vi "Scripted VI Path.vi"(7 "Terminal Descriptor":T1) -> (2 "Invalid?":bool, 3 "appended path":path)   [LabVIEW 2020, in "Parallel Diagram Block.xnode"]
uses:
  Parallel Diagram Block.xnode
  Parallel Block/Terminal Descriptor.ctl
  Parallel Block/Direction.ctl
  Parallel Block/Value Type.ctl
  Parallel Block/Terminal Type.ctl
  Parallel Block/Parallel Block.lvlib
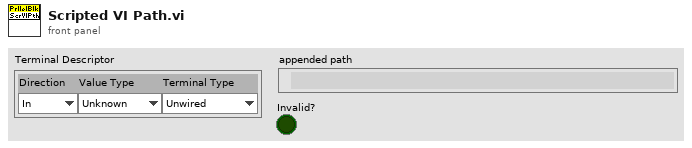
[diagram p1: front panel]
types:
  T1 = typedef "Parallel Block.lvlib/Terminal Descriptor.ctl" = cluster{"Direction":T2, "Value Type":T3, "Terminal Type":T4}
  T2 = typedef "Parallel Block.lvlib/Direction.ctl" = enum16{"In", "Out"}
  T3 = typedef "Parallel Block.lvlib/Value Type.ctl" = enum16{"Unknown", "Bool", "U8", "U16", "U32", "U64", "I8", "I16", "I32", "I64", "SGL", "DBL", "CSG", "CDB", "CDBWfm", "String", "DBLWfm"}
  T4 = typedef "Parallel Block.lvlib/Terminal Type.ctl" = enum16{"Unwired", "Connection", "Value", "Control Ref"}
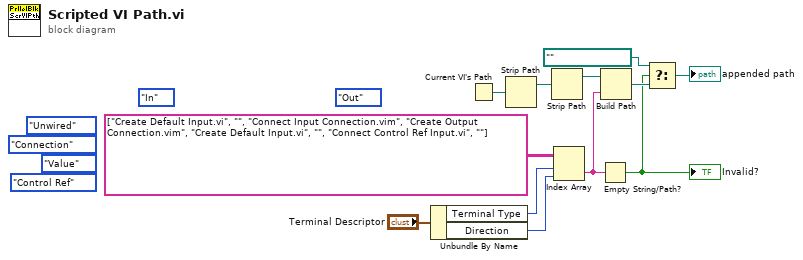
[diagram p0: block diagram]
diagram:
  (unwired) Direction."Out" ("Direction")
  (unwired) Direction."In" ("Direction")
  (unwired) Terminal_Type."Control Ref" ("Terminal Type")
  (unwired) Terminal_Type."Value" ("Terminal Type")
  (unwired) Terminal_Type."Connection" ("Terminal Type")
  (unwired) Terminal_Type."Unwired" ("Terminal Type")
  n1 = Unbundle By Name("Terminal Descriptor") -> ("Terminal Type"=w10:T4, "Direction"=w9:T2)
  n2 = Current VI's Path() -> (path=w8:path)
  n3 = Strip Path(path=w8) -> (stripped path=w7:path)  [unwired: 1 out]
  n4 = Strip Path(path=w7) -> (stripped path=w6:path)  [unwired: 1 out]
  n5 = Index Array(array=string[][] [["Create Default Input.vi", ""], ["Connect Input Connection.vim", "Create Output Connection.vim"], ["Create Default Input.vi", ""], ["Connect Control Ref Input.vi", ""]], index (row)=w10, index (col)=w9) -> (element=w5:string)
  n6 = Empty String/Path?(string/path=w5) -> (empty?=w2:bool)
  "Invalid?" <- w2
  n7 = Build Path(base path=w6, name or relative path=w5) -> (appended path=w4:path)
  n8 = Select(t=path "", s=w2, f=w4) -> (s? t:f=→"appended path":path)
